vi "AllDevicesAcquisitionRate.vi"(10 "Expt name":string="Bella", 11 "stop":refnum<vi>) -> (3 "status":string="running")   [LabVIEW 2020]
uses:
  Bella center GUIs/StagingBeamline/Controls/diagnosticQuee.ctl
  Shared/MySQL/Preset Query Enum.ctl
  Bella center GUIs/StagingBeamline/Controls/comunicationQueuecluster.ctl
  Bella center GUIs/StagingBeamline/Controls/stopQue.ctl
  Bella center GUIs/StagingBeamline/Controls/PingQueueTypDef.ctl
  Bella center GUIs/StagingBeamline/Controls/deviceQueue.ctl
panel:
  out "All devices status":T1(array[cluster]) {"Time (ms)" scale=0.0..5000.0}
  out "error history":string[](array[string])
  in  "Stop":bool=TRUE
  # "Bar max is 5 seconds"
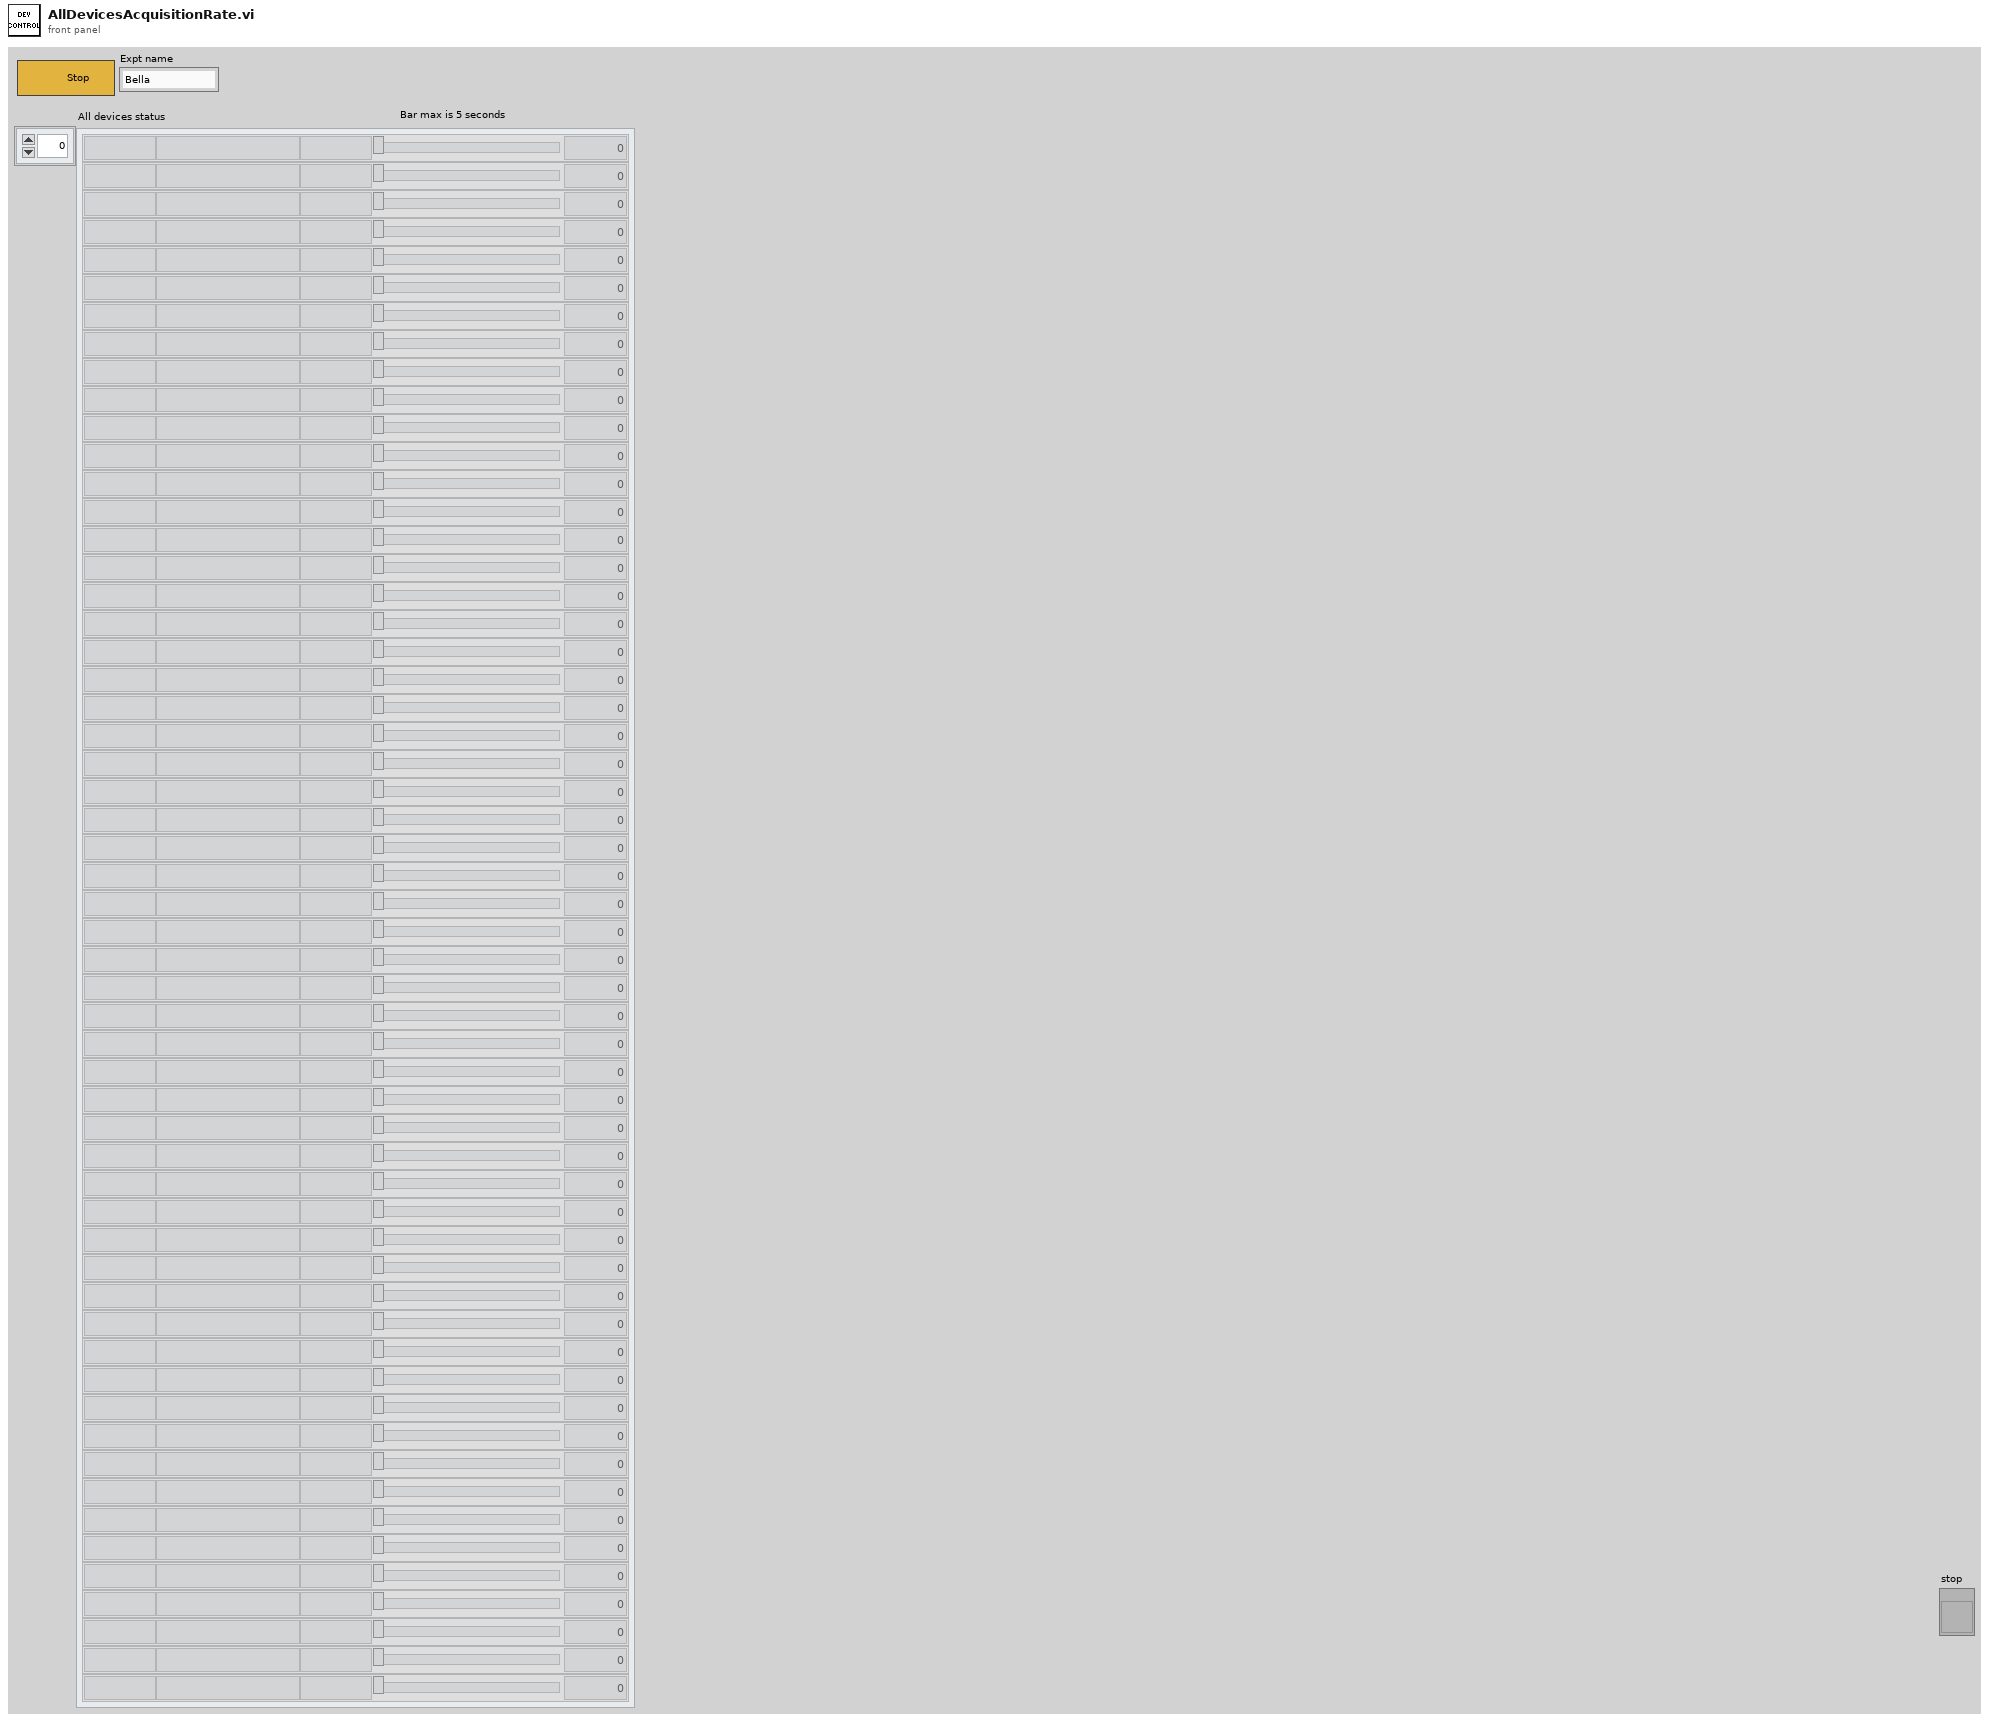
[diagram p1: front panel]
types:
  T1 = cluster{"Status":string, "Dev name":string, "Error":string, "Time (ms)":dbl, "time (ms) decimal":dbl}[]
  T2 = typedef "deviceQueue.ctl" = cluster{"device":string[], "XY Graph":cluster{"x":u32[], "Ramp Pattern":dbl[]}, "ststus":string[], "error":string[], "error history":string[]}
  T3 = typedef "PingQueueTypDef.ctl" = cluster{"Computers not on":string[]}
  T4 = typedef "stopQue.ctl" = cluster{"stop":bool}
  T5 = typedef "comunicationQueuecluster.ctl" = cluster{"device":string, "error history":string, "stop":bool}
  T6 = typedef "Preset Query Enum.ctl" = enum16{"Get Locations", "Get all IPs and MACs", "Get classes", "Get expt variables to set at scanstart for particular device", "Get expt devices and variables with start values", "Get expt devices and variables (with data to get)", "Get expt devices with data to get", "Get Expt devices and GUIs", "Get all devices basic properties", "Get Virtual Devices Core Info", "Get Expt names", "Get experiment basic properties", "Get experiment alarm variables", "Get MC Ports", "Get device network comm port", "Get devicetype lvclass path", "Get basic device properties", "Get Init Order", "Get all setable variables of a device", "Get device variable aliases", "Get force values of all settable variables", "Get all variables of a devicetype", "Get all variables of a device", "Get plotter details", "Get Saved Scans", "Get Scan Info", "GetGeneralGUIs", "Get expt for plotter", "Get plotter IDs from expt", "Get all devices", "Get all Virtual Devices", "Get all aliases", "Get variable and device info for Virtual Device", "GetItemLocatorIP", "Get IPs for GUIs", "Get DeviceType from Device", "GetLocalPortRange", "GetDevicePresetVariables", "Get Device Configuration", "GetAllPresetNames", "GetAllConfigurationNames", "GetPresetDeviceNames", "GetDeviceAliases", "GetDevicesOfClass"}
  T7 = typedef "diagnosticQuee.ctl" = cluster{"device":string[], "error":string[], "ststus":string[], "timing graph":cluster{u32[], "Ramp Pattern":dbl[]}, "error boolean":bool[], "error history":string[]}
  T8 = cluster{"Status":string, "Dev name":string, "Error":string, "Time (ms)":dbl, "time (ms) decimal":dbl}
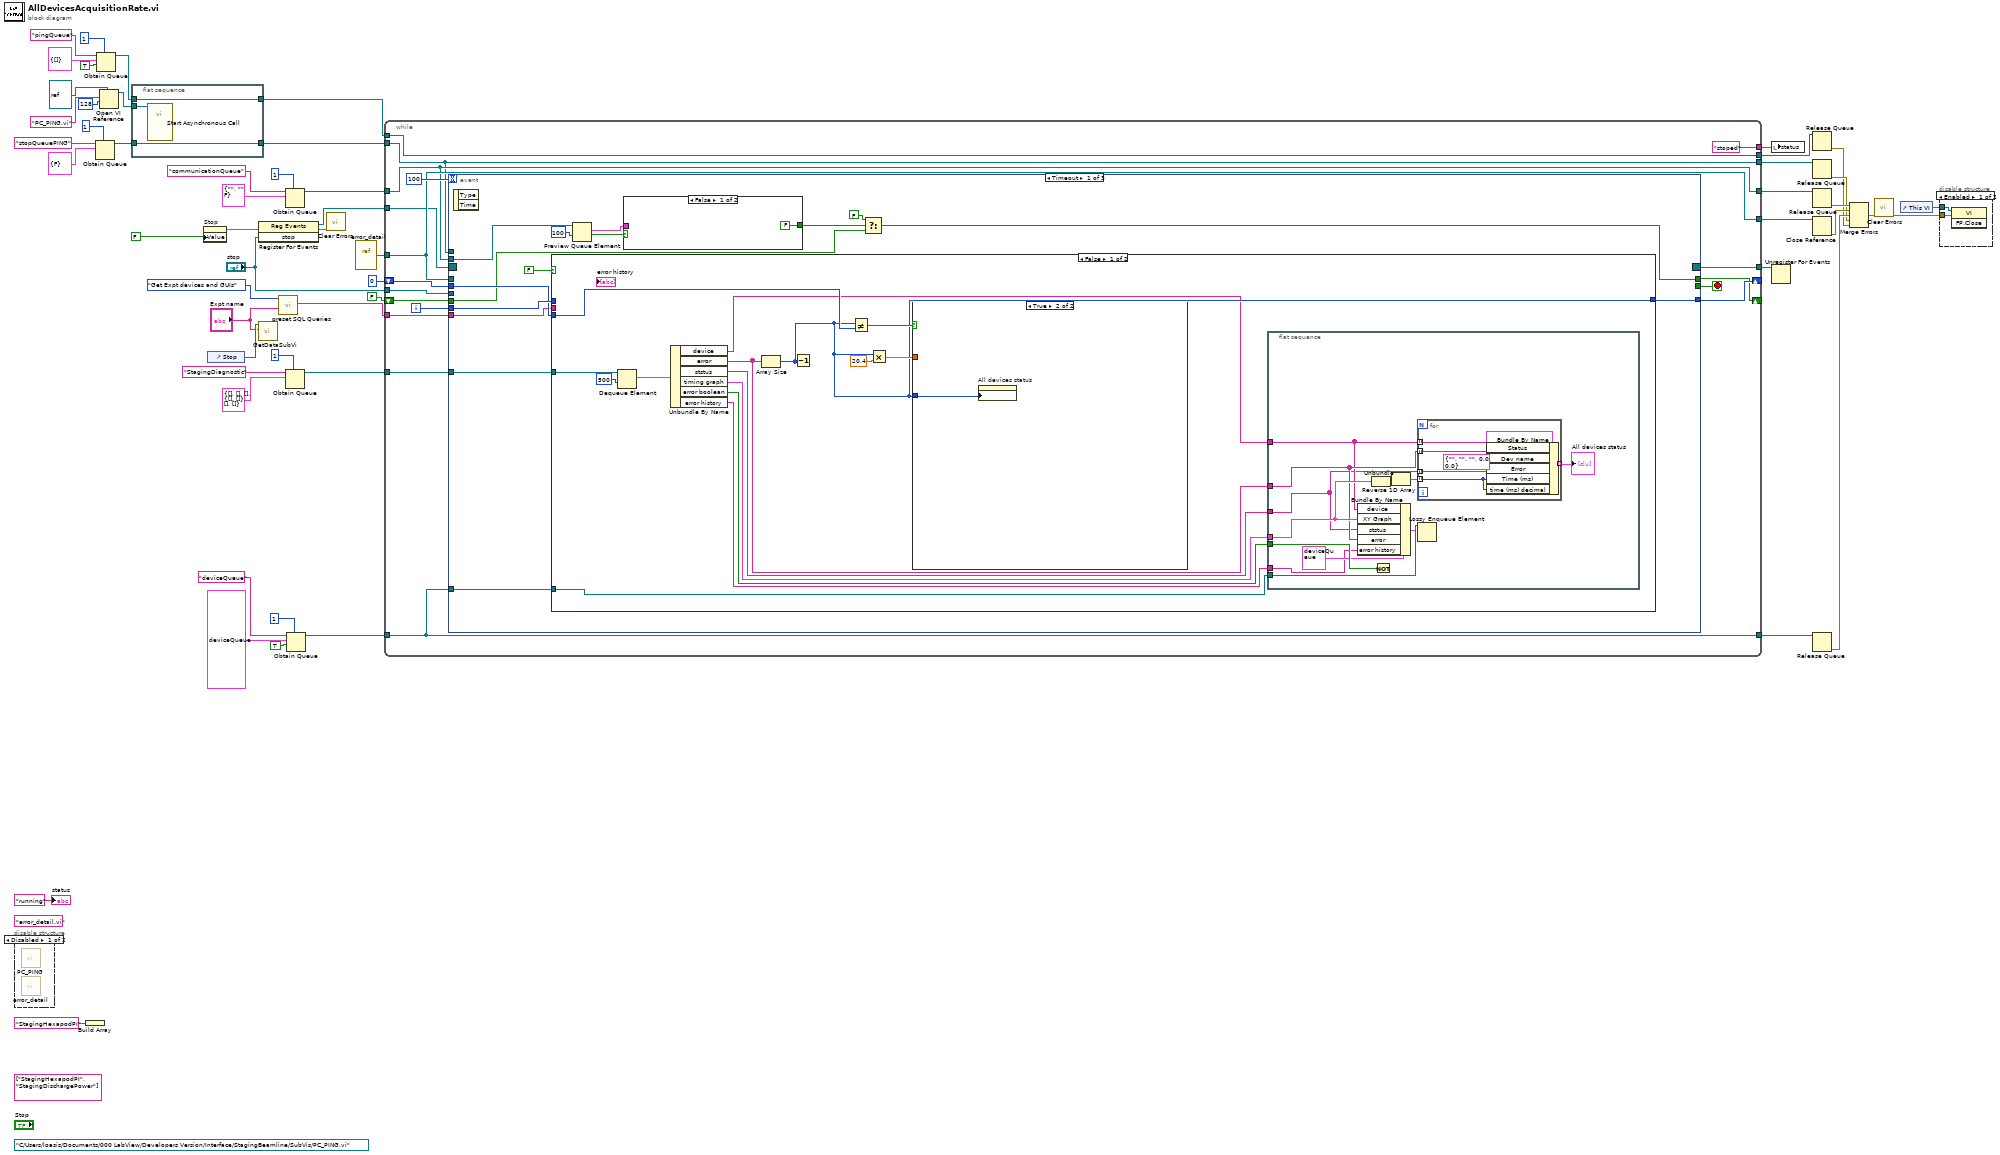
[diagram p0: block diagram]
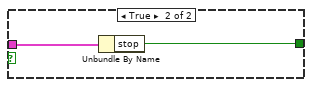
[diagram p4: hidden frame]
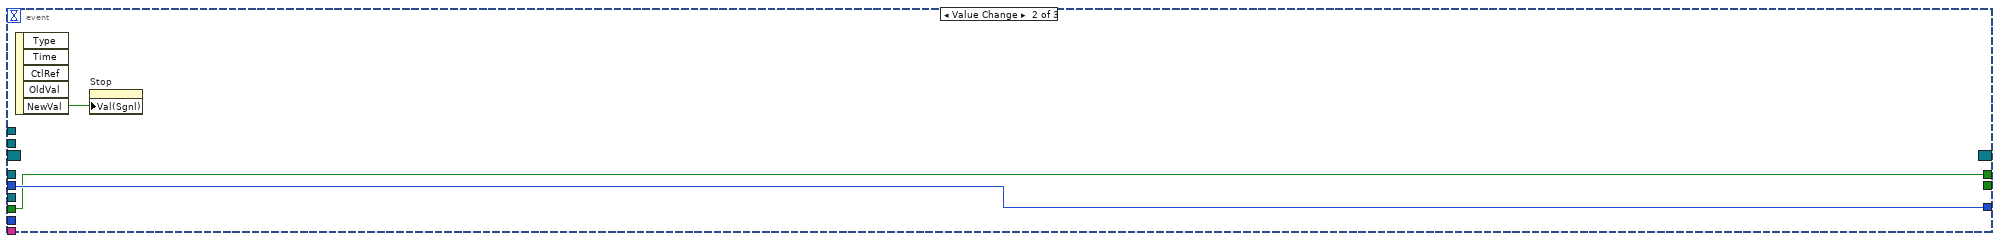
[diagram p7: hidden frame]
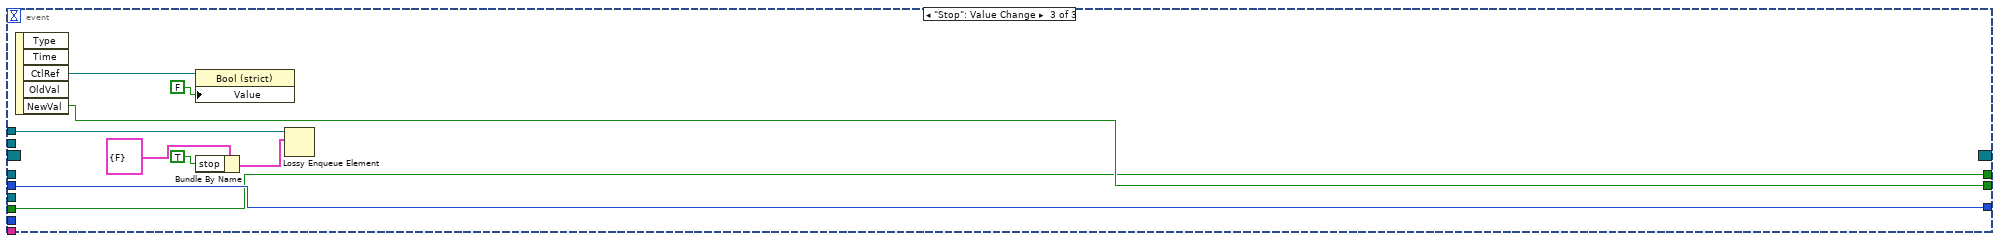
[diagram p8: hidden frame]
diagram:
  (unwired) "error_detail.vi" ("name (unnamed)")
  (unwired) path "C:/Users/loasis/Documents/000 LabView/Developers Version/Interface/StagingBeamline/SubVis/PC_PING.vi" ("vi path")
  (unwired) string[] ["StagingHexapodPI", "StagingDischargePower"]
  n1 = disable-structure shown="Disabled" {
    frame Disabled {
      n2 = call "PC_PING.vi"() -> ()  [unwired: 12 in]
      n3 = call "error_detail.vi"() -> ()  [unwired: 12 in]
    }
    frame Enabled {
    }
  }
  n4 = Build Array("StagingHexapodPI" ("String")) -> ()  [unwired: 1 out]
  n5 = Obtain Queue(max queue size (-1, unlimited)=1, name (unnamed)="stopQueuePING", element data type=T4 {"stop"=FALSE}) -> (queue out=w25:refnum<queue>)  [unwired: 2 in, 2 out]
  n6 = Obtain Queue(max queue size (-1, unlimited)=1, name (unnamed)="pingQueue", element data type=T3 {"Computers not on"=[]}, create if not found? (T)=TRUE) -> (queue out=w27:refnum<queue>)  [unwired: 1 in, 2 out]
  n7 = Open VI Reference(type specifier VI Refnum (for type only)=refnum<vi> refnum, vi path="PC_PING.vi" ("name (unnamed)"), options=128) -> (vi reference=w21:refnum<vi>)  [unwired: 3 in, 1 out]
  n8 = flat-sequence {
    tunnel: w27 -> [w60]
    tunnel: [w60] -> w26
    tunnel: w25 -> [w59]
    tunnel: [w59] -> w24
    tunnel: w21 -> [w58]
    frame #0 {
      n9 = call-by-ref "Start Asynchronous Call"(reference=w58) -> ()  [unwired: 13 in, 2 out]
    }
  }
  n10 = property on="Stop" class="Bool (strict)"("Value"=FALSE) -> (error out=w4:errorcluster)  [unwired: 2 in, 1 out]
  n11 = control-ref of="Stop"() -> (w54:refnum<vi>)
  n12 = register-events(error in=w4, "stop") -> (reference out=w11:refnum<event-registration>, error out=w5:errorcluster)  [unwired: 1 in]
  n13 = call "GetDataSubVi.vi"("Expt name"="Expt name", "Stop 2"=w54) -> ()  [unwired: 10 in]
  n14 = call "preset SQL Queries.vi"("Expt name / MCIP/ Variable/Preset Name"="Expt name", "Preset Query"=Preset_Query_Enum."Get Expt devices and GUIs") -> ("1st column 1st data"=w55:string[])  [unwired: 7 in, 2 out]
  n15 = Obtain Queue(max queue size (-1, unlimited)=1, name (unnamed)="communicationQueue", element data type=T5 {"device"="", "error history"="", "stop"=FALSE}) -> (queue out=w44:refnum<queue>)  [unwired: 2 in, 2 out]
  n16 = Obtain Queue(max queue size (-1, unlimited)=1, name (unnamed)="StagingDiagnostic", element data type=T7 {"device"=[], "error"=[], "ststus"=[], "timing graph"={[], "Ramp Pattern"=[]}, "error boolean"=[], "error history"=[]} ("output cluster")) -> (queue out=w50:refnum<queue>)  [unwired: 2 in, 2 out]
  n17 = Obtain Queue(max queue size (-1, unlimited)=1, name (unnamed)="deviceQueue", element data type=T2 {"device"=["StagingM1Far", "StagingM1Near", "StagingM3Far", "StagingM5", "StagingOAP2Near", "StagingOAP1Near", "StagingPXISlow", "StagingOAP2Far", "StagingLowPressure1", "StagingHexapodPI", "StagingDG645_1", "StagingLowPressure2", "StagingPXIFast2", "StagingPXIFast1", "StagingAlignBeam1", "StagingAlignBeam2", "StagingFilterWheels", "StagingShotControl", "StagingDG645_2", "StagingTRA3", "StagingGuppy", "TREX PXI fast", "StagingNISwitch", "StagingEnergy", "StagingTelescopePosition", "StagingDischargePower", "StagingDischargeHV", "StagingInterlock", "StagingAnalysisSlow", "Staging1Wire", "StagingTRA2", "StagingTelescopeImageLocation", "StagingBeam1OAPMotors", "StagingM4", "StagingDelayStage", "StagingTRA1", "StagingOAP1Far", "StagingFocusPositionBeam1", "StagingFocusPositionBeam2", "TREX TRA1", "StagingHighPressureDAQ", "StagingHighPressureController"], "XY Graph"={"x"=[154, 10000, 41, 80, 72, 7, 151, 45, 108, 239, 223, 116, 0, 109, 143, 4, 112, 224, 106, 57, 89, 58, 39, 40, 414, 148, 167, 127, 199, 314, 183, 174, 107, 5, 104, 505, 42, 76, 44, 102, 3, 30], "Ramp Pattern"=[0.0, 1.0, 2.0, 3.0, 4.0, 5.0, 6.0, 7.0, 8.0, 9.0, 10.0, 11.0, 12.0, 13.0, 14.0, 15.0, 16.0, 17.0, 18.0, 19.0, 20.0, 21.0, 22.0, 23.0, 24.0, 25.0, 26.0, 27.0, 28.0, 29.0, 30.0, 31.0, 32.0, 33.0, 34.0, 35.0, 36.0, 37.0, 38.0, 39.0, 40.0, 41.0]}, "ststus"=["Initialized", "Initialized", "Initialized", "Initialized", "Initialized", "Initialized", "Initialized", "Initialized", "Initialized", "Initialized", "Initialized", "Initialized", "Initialized", "Initialized", "Initialized", "Initialized", "Initialized", "Initialized", "Initialized", "Initialized", "Initialized", "Initialized", "Initialized", "Initialized", "Initialized", "Initialized", "Initialized", "Initialized", "Initialized", "Initialized", "Initialized", "Initialized", "Initialized", "Initialized", "Initialized", "Initialized", "Initialized", "Initialized", "Initialized", "Initialized", "no response", "Initialized"], "error"=["no error", "no error", "no error", "error", "no error", "no error", "no error", "no error", "no error", "no error", "no error", "no error", "no error", "no error", "no error", "no error", "no error", "no error", "no error", "no error", "error", "no error", "no error", "no error", "no error", "no error", "no error", "no error", "no error", "no error", "no error", "no error", "no error", "no error", "no error", "no error", "no error", "no error", "no error", "no error", "no response", "no error"], "error history"=[]} ("deviceQueue"), create if not found? (T)=TRUE) -> (queue out=w29:refnum<queue>)  [unwired: 1 in, 2 out]
  n18 = call <vilib>:"Clear Errors.vi"("error in (no error)"=w5) -> ()  [unwired: 5 in, 2 out]
  n19 = vi-ref "error_detail.vi"() -> (w1:refnum<vi>)
  n20 = while {
    tunnel: w55 -> [w75]
    shift-right: [w74] -> _
    shift-left: u32 0 ("Number of Rows") -> [w73]
    tunnel: w50 -> [w72]
    tunnel: w1 -> [w71]
    tunnel: [w71] -> w48
    shift-right: [w69] -> _
    shift-left: FALSE -> [w70]
    tunnel: w44 -> [w68]
    tunnel: [w68] -> w43
    tunnel: w24 -> [w67]
    tunnel: [w67] -> w39
    tunnel: w26 -> [w66]
    tunnel: [w66] -> w34
    tunnel: w29 -> [w65]
    tunnel: [w65] -> w28
    tunnel: w11 -> [w64]
    tunnel: [w63] -> w10
    tunnel: ["stoped"] -> w8
    tunnel: "stop" -> [w61]
    i -> [w76]
    stop <- w78 stop-if-true
    n21 = event shown="[0] Timeout" {
      selector: w64 -> [_ _ _]
      dyn-events: [_ _ _] -> w63
      timeout: 100 -> [_ _ _]
      tunnel: [_ _ w143] -> w78
      tunnel: w76 -> [w93 _ _]
      tunnel: w75 -> [w90 _ _]
      tunnel: [w92 w134 w142] -> w74
      tunnel: w73 -> [w91 w134 w142]
      tunnel: w72 -> [w89 _ _]
      tunnel: w71 -> [_ _ _]
      tunnel: w70 -> [w82 w133 w139]
      tunnel: [w83 w133 w139] -> w69
      tunnel: w68 -> [w86 _ _]
      tunnel: w67 -> [_ _ w138]
      tunnel: w65 -> [w87 _ _]
      tunnel: w61 -> [_ _ _]
      event Timeout {
        n22 = event-data() -> ()  [unwired: 1 in, 2 out]
        n23 = case shown="False" FALSE {
          tunnel: w93 -> [_ _]
          tunnel: w90 -> [_ _]
          tunnel: [w107 w131] -> w92
          tunnel: w91 -> [w109 w131]
          tunnel: w89 -> [w106 _]
          tunnel: w87 -> [w98 _]
          frame False {
            n24 = Dequeue Element(queue=w106, timeout in ms (-1)=500) -> (element=w105:T7)  [unwired: 1 in, 3 out]
            n25 = Unbundle By Name(w105) -> ("device"=w100:string[], "error"=w101:string[], "ststus"=w103:string[], "timing graph"=w104:cluster{u32[], "Ramp Pattern":dbl[]}, "error boolean"=w102:bool[], "error history"=w97:string[])
            n26 = Array Size(array=w101) -> (size(s)=w107:i32)
            n27 = Decrement(x=w107) -> ()  [unwired: 1 out]
            n28 = Not Equal?(x=w107, y=w109) -> (x != y?=w108:bool)
            n29 = Multiply(x=w107, y=20.4) -> (x*y=w110:dbl)
            n30 = case shown="True" w108 {
              tunnel: w107 -> [_ w112]
              tunnel: w110 -> [_ _]
              frame False {
              }
              frame True {
                n31 = property on="All devices status" class="Arr (strict)"("Number of Rows"=w112) -> ()  [unwired: 2 in, 2 out]
              }
            }
            n32 = flat-sequence {
              tunnel: w104 -> [w119]
              tunnel: w103 -> [w115]
              tunnel: w102 -> [w124]
              tunnel: w101 -> [w117]
              tunnel: w100 -> [w116]
              tunnel: w98 -> [w123]
              tunnel: w97 -> [w120]
              frame #0 {
                n33 = Bundle By Name(cluster=T2 {"device"=["StagingM1Far", "StagingM1Near", "StagingM3Far", "StagingM5", "StagingOAP2Near", "StagingOAP1Near", "StagingPXISlow", "StagingOAP2Far", "StagingLowPressure1", "StagingHexapodPI", "StagingDG645_1", "StagingLowPressure2", "StagingPXIFast2", "StagingPXIFast1", "StagingAlignBeam1", "StagingAlignBeam2", "StagingFilterWheels", "StagingShotControl", "StagingDG645_2", "StagingTRA3", "StagingGuppy", "TREX PXI fast", "StagingNISwitch", "StagingEnergy", "StagingTelescopePosition", "StagingDischargePower", "StagingDischargeHV", "StagingInterlock", "StagingAnalysisSlow", "Staging1Wire", "StagingTRA2", "StagingTelescopeImageLocation", "StagingBeam1OAPMotors", "StagingM4", "StagingDelayStage", "StagingTRA1", "StagingOAP1Far", "StagingFocusPositionBeam1", "StagingFocusPositionBeam2", "TREX TRA1", "StagingHighPressureDAQ", "StagingHighPressureController"], "XY Graph"={"x"=[154, 10000, 41, 80, 72, 7, 151, 45, 108, 239, 223, 116, 0, 109, 143, 4, 112, 224, 106, 57, 89, 58, 39, 40, 414, 148, 167, 127, 199, 314, 183, 174, 107, 5, 104, 505, 42, 76, 44, 102, 3, 30], "Ramp Pattern"=[0.0, 1.0, 2.0, 3.0, 4.0, 5.0, 6.0, 7.0, 8.0, 9.0, 10.0, 11.0, 12.0, 13.0, 14.0, 15.0, 16.0, 17.0, 18.0, 19.0, 20.0, 21.0, 22.0, 23.0, 24.0, 25.0, 26.0, 27.0, 28.0, 29.0, 30.0, 31.0, 32.0, 33.0, 34.0, 35.0, 36.0, 37.0, 38.0, 39.0, 40.0, 41.0]}, "ststus"=["Initialized", "Initialized", "Initialized", "Initialized", "Initialized", "Initialized", "Initialized", "Initialized", "Initialized", "Initialized", "Initialized", "Initialized", "Initialized", "Initialized", "Initialized", "Initialized", "Initialized", "Initialized", "Initialized", "Initialized", "Initialized", "Initialized", "Initialized", "Initialized", "Initialized", "Initialized", "Initialized", "Initialized", "Initialized", "Initialized", "Initialized", "Initialized", "Initialized", "Initialized", "Initialized", "Initialized", "Initialized", "Initialized", "Initialized", "Initialized", "no response", "Initialized"], "error"=["no error", "no error", "no error", "error", "no error", "no error", "no error", "no error", "no error", "no error", "no error", "no error", "no error", "no error", "no error", "no error", "no error", "no error", "no error", "no error", "error", "no error", "no error", "no error", "no error", "no error", "no error", "no error", "no error", "no error", "no error", "no error", "no error", "no error", "no error", "no error", "no error", "no error", "no error", "no error", "no response", "no error"], "error history"=[]} ("deviceQueue"), "device"=w116, "XY Graph"=w119, "ststus"=w115, "error"=w117, "error history"=w120) -> (w121:T2)
                n34 = Unbundle(w119) -> (w118:u32[])  [unwired: 1 out]
                n35 = Not(x=w124) -> ()  [unwired: 1 out]
                n36 = Reverse 1D Array(array=w118) -> (reversed array=w113:u32[])
                n37 = for {
                  tunnel: [w130] -> w114 mode=indexing
                  tunnel: w113 -> [w125] mode=indexing
                  tunnel: w117 -> [w129] mode=indexing
                  tunnel: w116 -> [w128] mode=indexing
                  tunnel: w115 -> [w127] mode=indexing
                  n38 = Bundle By Name(cluster=T8 {"Status"="", "Dev name"="", "Error"="", "Time (ms)"=0.0, "time (ms) decimal"=0.0} ("Device status"), "Status"=w127, "Dev name"=w128, "Error"=w129, "Time (ms)"=w125, "time (ms) decimal"=w125) -> (w130:T8)
                }
                "All devices status" <- w114
                n39 = Lossy Enqueue Element(queue=w123, element=w121) -> ()  [unwired: 1 in, 4 out]
              }
            }
          }
          frame True {
          }
        }
        n40 = Preview Queue Element(queue=w86, timeout in ms (-1)=100) -> (element=w85:T5, timed out?=w79:bool)  [unwired: 1 in, 2 out]
        n41 = case shown="False" w79 {
          tunnel: w85 -> [_ w96]
          tunnel: [FALSE w95] -> w84
          frame False {
          }
          frame True {
            n42 = Unbundle By Name(w96) -> ("stop"=w95:bool)
          }
        }
        n43 = Select(t=FALSE, s=w84, f=w82) -> (s? t:f=w83:bool)
      }
      event Value Change {
        n44 = event-data() -> ("NewVal"=w132:bool)  [unwired: 1 in, 4 out]
        n45 = property on="Stop" class="Bool (strict)"("Val(Sgnl)"=w132) -> ()  [unwired: 2 in, 2 out]
      }
      event "Stop": Value Change {
        n46 = event-data() -> ("CtlRef"=w141:refnum<vi>, "NewVal"=w143:bool)  [unwired: 1 in, 3 out]
        n47 = property class="Bool (strict)"(reference=w141, "Value"=FALSE) -> ()  [unwired: 1 in, 2 out]
        n48 = Bundle By Name(cluster=T4 {"stop"=FALSE}, "stop"=TRUE) -> (w135:T4)
        n49 = Lossy Enqueue Element(queue=w138, element=w135) -> ()  [unwired: 1 in, 4 out]
      }
    }
  }
  n50 = local write "status"(w8) -> ()
  n51 = Unregister For Events(event registration refnum=w10) -> ()  [unwired: 1 in, 1 out]
  n52 = Release Queue(queue=w34) -> (error out=w15:errorcluster)  [unwired: 2 in, 2 out]
  n53 = Release Queue(queue=w39) -> (error out=w16:errorcluster)  [unwired: 2 in, 2 out]
  n54 = Release Queue(queue=w43) -> (error out=w19:errorcluster)  [unwired: 2 in, 2 out]
  n55 = Close Reference(reference=w48) -> (error out=w18:errorcluster)  [unwired: 1 in]
  n56 = Release Queue(queue=w28) -> (error out=w17:errorcluster)  [unwired: 2 in, 2 out]
  n57 = Merge Errors(w19, w18, w17, w16, w15) -> (w14:errorcluster)
  n58 = call <vilib>:"Clear Errors.vi"("error in (no error)"=w14) -> ("error out"=w13:errorcluster)  [unwired: 5 in, 1 out]
  n59 = control-ref of="This VI"() -> (w12:refnum<vi>)
  n60 = disable-structure shown="Enabled" {
    disable-tunnel: w13 -> [w145 _]
    disable-tunnel: w12 -> [w144 _]
    frame Enabled {
      n61 = invoke class="VI" method="FP.Close"(reference=w144, error in=w145) -> ()  [unwired: 1 in, 3 out]
    }
    frame Disabled {
    }
  }
  "status" <- "running"
